vi "Get Path&PassFail from DVR.vi"(8 "error in (no error)":errorcluster, 11 "Data Value Reference in":T1) -> (0 "error out":errorcluster, 1 "FileName":string, 2 "CsvPath":path, 3 "Data Value Reference out":T1, 4 "Pass?":bool)   [LabVIEW 2011]
uses:
  Controls/DVR of CSV Tests Data.ctl
  Controls/CSVs Tests Data.ctl
  Controls/Test Column Data.ctl
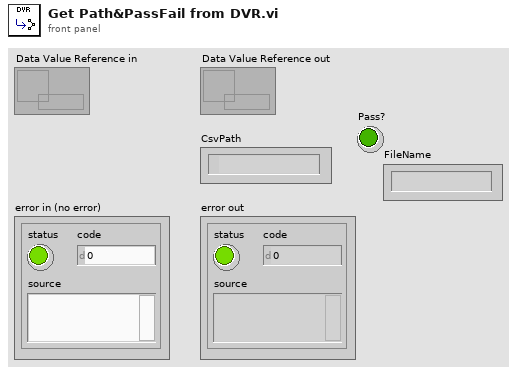
[diagram p1: front panel]
types:
  T1 = typedef "DVR of CSV Tests Data.ctl" = refnum<data-value>
  T2 = typedef "CSVs Tests Data.ctl" = cluster{"Test Data":T3[], "CsvPath":path, "LogPath":path, "Pass?":bool, "Error":errorcluster}
  T3 = typedef "Test Column Data.ctl" = cluster{"Chn":string, "ExpVals":dbl[], "TimeStamps":i64[], "NegTol":dbl, "PosTol":dbl}
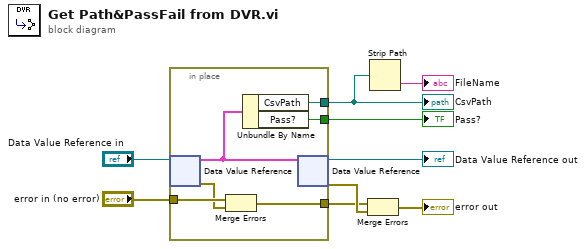
[diagram p0: block diagram]
diagram:
  n1 = in-place {
    in-place-border: "error in (no error)" -> [w15]
    in-place-border: [w12] -> w6
    in-place-border: [w11] -> w2
    in-place-border: [w10] -> w3
    n2 = in-place-dvr #1("Data Value Reference in") -> (w13:T2, w14:errorcluster)
    n3 = Merge Errors(w15, w14) -> (w12:errorcluster)
    n4 = Unbundle By Name(w13) -> ("CsvPath"=w11:path, "Pass?"=w10:bool)
    n5 = in-place-dvr #1(w13) -> (→"Data Value Reference out":T1, w7:errorcluster)
  }
  "CsvPath" <- w2
  "Pass?" <- w3
  n6 = Merge Errors(w6, w7) -> (→"error out":errorcluster)
  n7 = Strip Path(path=w2) -> (name=→"FileName":string)  [unwired: 1 out]
